vi "oa_Concatenate Even Angle Signal and Trigger Indices (1 Channel).vi"(7 "reset?":bool, 8 "history trigger indices":T1, 9 "trigger indices":T1, 10 "history even angle signal":cluster{"r0":dbl, "dr":dbl, "Y":dbl[]}={"r0"=0.0, "dr"=1.0, "Y"=[]} {"r0" format="%.2p"; "dr" format="%.2p"; "Y" format="%.2f"}, 11 "even angle signal":cluster{"r0":dbl, "dr":dbl, "Y":dbl[]}={"r0"=0.0, "dr"=1.0, "Y"=[]} {"r0" format="%.2p"; "dr" format="%.2p"; "Y" format="%.2f"}) -> (1 "trigger indices out":T1, 3 "even angle signal out":cluster{"r0":dbl, "dr":dbl, "Y":dbl[]}={"r0"=0.0, "dr"=1.0, "Y"=[]} {"r0" format="%.2p"; "dr" format="%.2p"; "Y" format="%.2f"})   [LabVIEW 2017, in "SoundVib_OAUtility.lvlib"]
uses:
  <vilib>/addons/Sound and Vibration/Order Analysis/Utility/SoundVib_OAUtility.lvlib
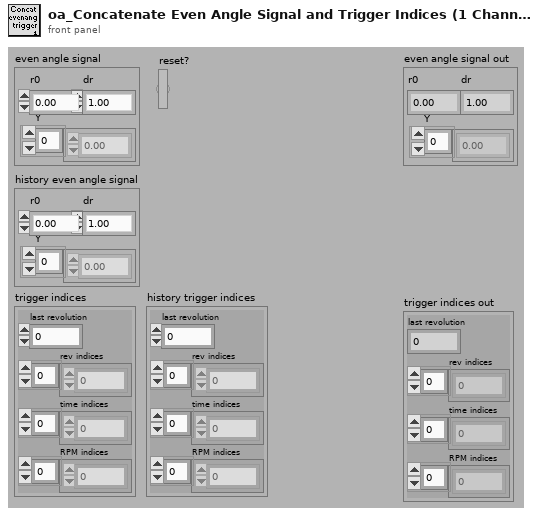
[diagram p1: front panel]
types:
  T1 = cluster{"last revolution":dbl, "rev indices":dbl[], "time indices":dbl[], "RPM indices":dbl[]}
  T2 = cluster{"last revolution":dbl, dbl[], dbl[], dbl[]}
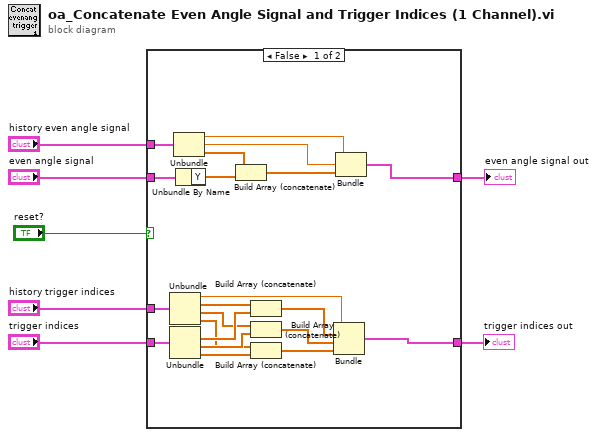
[diagram p0: block diagram]
diagram:
  n1 = case shown="False" "reset?" {
    tunnel: "even angle signal" -> [w27 w30]
    tunnel: [w21 w30] -> w5
    tunnel: "trigger indices" -> [w20 w29]
    tunnel: [w8 w29] -> w3
    tunnel: "history even angle signal" -> [w28 _]
    tunnel: "history trigger indices" -> [w19 _]
    frame False {
      n2 = Unbundle(w19) -> ("last revolution"=w9:dbl, "rev indices"=w18:dbl[], "time indices"=w16:dbl[], "RPM indices"=w14:dbl[])
      n3 = Unbundle(w20) -> ("rev indices"=w17:dbl[], "time indices"=w15:dbl[], "RPM indices"=w13:dbl[])  [unwired: 1 out]
      n4 = Unbundle(w28) -> ("r0"=w24:dbl, "dr"=w23:dbl, "Y"=w26:dbl[])
      n5 = Unbundle By Name(w27) -> ("Y"=w25:dbl[])
      n6 = Build Array (concatenate)(w26, w25) -> (w22:dbl[])
      n7 = Build Array (concatenate)(w18, w17) -> (w12:dbl[])
      n8 = Build Array (concatenate)(w16, w15) -> (w11:dbl[])
      n9 = Build Array (concatenate)(w14, w13) -> (w10:dbl[])
      n10 = Bundle("last revolution"=w9, w12, w11, w10) -> (w8:T2)  [unwired: 1 in]
      n11 = Bundle("r0"=w24, "dr"=w23, w22) -> (w21:cluster{"r0":dbl, "dr":dbl, dbl[]})  [unwired: 1 in]
    }
    frame True {
    }
  }
  "even angle signal out" <- w5
  "trigger indices out" <- w3
